vi "GetAxisIndex.vi"(8 "error in (no error)":errorcluster, 10 "axis name":string, 11 "controller in":refnum<k24>) -> (0 "error out":errorcluster, 2 "axis index":i32, 3 "controller out":refnum<k24>)   [LabVIEW 2016]
uses:
  C:/user/patrick/git/Aerotech-Delay-Line/lvsrc/Aerotech-Ensemble-LabVIEW/8.2/Bin/Aerotech.Ensemble.dll
  Bin/Aerotech.Ensemble.dll
  C:/user/patrick/git/Aerotech-Delay-Line/lvsrc/Aerotech-Ensemble-LabVIEW/8.2/Bin/Aerotech.Ensemble.LabVIEW.dll
  Bin/Aerotech.Ensemble.LabVIEW.dll
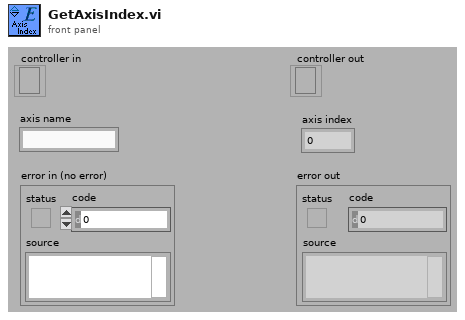
[diagram p1: front panel]
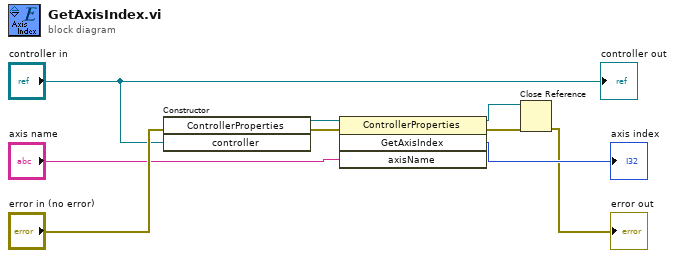
[diagram p0: block diagram]
diagram:
  n1 = constructor class="ControllerProperties"(error in="error in (no error)", "controller"="controller in") -> (reference out=w7:refnum<k24>, error out=w6:errorcluster)  [unwired: 2 in, 2 out]
  n2 = invoke class="ControllerProperties" method="GetAxisIndex"(reference=w7, error in=w6, "axisName"="axis name") -> (reference out=w3:refnum<k24>, error out=w2:errorcluster, "GetAxisIndex"=→"axis index":i32)  [unwired: 1 in, 1 out]
  n3 = Close Reference(reference=w3, error in (no error)=w2) -> (error out=→"error out":errorcluster)
  "controller out" <- "controller in"
